vi "File1.vi"() -> ()   [LabVIEW 2019]
uses:
  <vilib>/measure/NI_MABase.lvlib
panel:
  in  "Fvz":dbl
  out "Numeric":i32
  in  "stop":bool
  in  "Sirka okna (ms)":i32(listbox)
  out "Waveform Graph":waveform(dbl)(graph)
  in  "Offset":dbl format="%0.2p"
  in  "Faze":dbl format="%.2p"
  in  "Amplituda":dbl=1.0 format="%0.2p"
  in  "Frekvence":dbl=10.0 format="%0.2p"
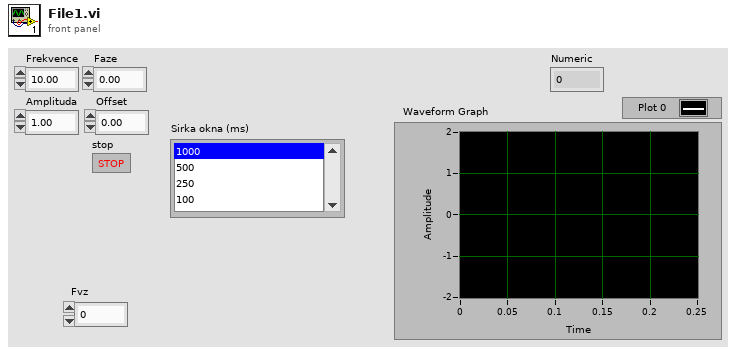
[diagram p1: front panel]
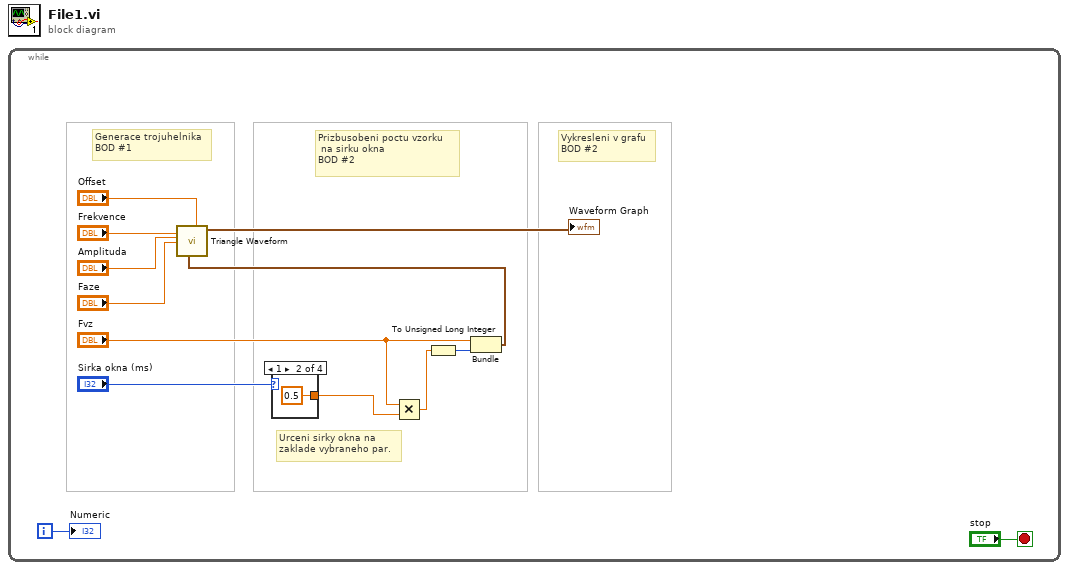
[diagram p0: block diagram]
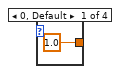
[diagram p2: hidden frame]
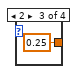
[diagram p3: hidden frame]
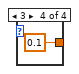
[diagram p4: hidden frame]
diagram:
  n1 = while {
    i -> [w8]
    stop <- "stop" stop-if-true
    # "Urceni sirky okna na\nzaklade vybraneho par."
    # "Prizbusobeni poctu vzorku\n na sirku okna\nBOD #2"
    # "Vykresleni v grafu\nBOD #2"
    # "Generace trojuhelnika\nBOD #1"
    n2 = case shown="1" "Sirka okna (ms)" {
      tunnel: [1.0 ("X Scale.Range:Maximum") 0.5 ("X Scale.Range:Maximum") 0.25 ("X Scale.Range:Maximum") 0.1 ("X Scale.Range:Maximum")] -> w5
      frame 0, Default {
      }
      frame 1 {
      }
      frame 2 {
      }
      frame 3 {
      }
    }
    n3 = Multiply(x="Fvz", y=w5) -> (x*y=w1:dbl)
    n4 = To Unsigned Long Integer(number=w1) -> (unsigned 32bit integer=w2:u32)
    n5 = Bundle("Fvz"="Fvz", w2) -> (w3:cluster{"Fvz":dbl, u32})  [unwired: 1 in]
    n6 = call <vilib>:"Triangle Waveform.vi"("offset"="Offset", "sampling info"=w3, "phase"="Faze", "amplitude"="Amplituda", "frequency"="Frekvence") -> ("signal out"=→"Waveform Graph":waveform(dbl))  [unwired: 5 in, 1 out]
    "Numeric" <- w8
  }
